vi "DMA Write-FPGA.vi"() -> ()   [LabVIEW 2012]
uses:
  <vilib>/rvi/eio/common/nirviEmuTemplateMethod_errors.vi
  <vilib>/rvi/interface/RandomDataEmulation/nirviRandomDataFPGAFIFO.vi
  <vilib>/rvi/interface/RandomDataEmulation/niFpgaRandomDataHandleErrors.vi
  <vilib>/rvi/Emulation/niFpgaSctlEmulationGetInTimedLoop.vi
  <vilib>/rvi/Emulation/niFpgaSctlEmulationGlobalWrite.vi
  <vilib>/eio/EIONode/EIONode.xnode
  <vilib>/rvi/DataTransferAndStorage/Container/XNode/niFpgaContainer.xnode
  <vilib>/rvi/interface/RandomDataEmulation/nirviRandomDataFpgaReadWriteTemplate.vi
panel:
  out "Overflow?":bool
  in  "Count(us)":u32=4000
  in  "DMA Cleared?":bool
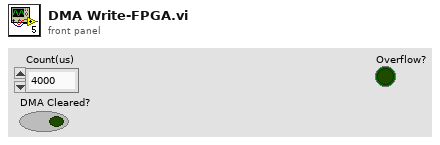
[diagram p1: front panel]
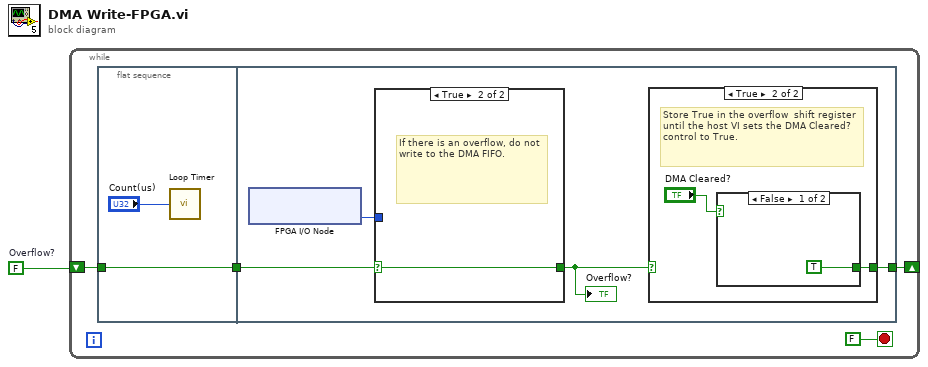
[diagram p0: block diagram]
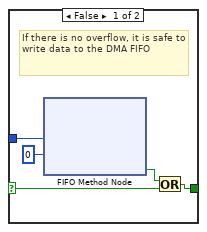
[diagram p2: hidden frame]
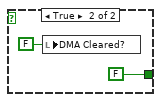
[diagram p4: hidden frame]
diagram:
  w1 = FALSE  # Overflow?
  n1 = while {
    shift-right: [w3] -> _
    shift-left: w1 -> [w4]
    stop <- FALSE stop-if-true
    n2 = flat-sequence {
      tunnel: w4 -> [w7]
      tunnel: [w7] -> w2
      tunnel: [w9] -> w3
      tunnel: w2 -> [w11]
      frame #0 {
        n3 = call "Loop Timer"("Count(uSec)"="Count(us)") -> ()  [unwired: 1 out]
      }
      frame #1 {
        n4 = xnode "FPGA I/O Node"() -> ("Analog Input"=w8:i16)  [unwired: 1 in, 1 out]
        n5 = case shown="True" w11 {
          selector: w11 -> [w13 w17]
          tunnel: [w15 w17] -> w10
          tunnel: w8 -> [w14 _]
          frame False {
            # "If there is no overflow, it is safe to write data to the DMA FIFO"
            n6 = xnode "FIFO Method Node"("Element"=w14, "Timeout"=0) -> ("Timed Out?"=w16:bool)  [unwired: 1 in, 1 out]
            n7 = Or(x=w16, y=w13) -> (x .or. y?=w15:bool)
          }
          frame True {
            # "If there is an overflow, do not write to the DMA FIFO."
          }
        }
        "Overflow?" <- w10
        n8 = case shown="True" w10 {
          selector: w10 -> [w18 _]
          tunnel: [w18 w19] -> w9
          frame False {
          }
          frame True {
            # "Store True in the overflow  shift register until the host VI sets the DMA Cleared? control to True."
            n9 = case shown="False" "DMA Cleared?" {
              tunnel: [TRUE FALSE] -> w19
              frame False {
              }
              frame True {
                n10 = local write "DMA Cleared?"(FALSE ("Reset")) -> ()
              }
            }
          }
        }
      }
    }
  }
